vi "Vision Processing.vi"(4 "error in (no error)":errorcluster, 6 "CameraDevRef":T1) -> ()   [LabVIEW 2011]
uses:
  <vilib>/Rock Robotics/WPI/Camera/WPI_CameraDevRef.ctl
  Robot Global Data.vi
  <vilib>/vision/NI_Vision_Development_Module.lvlib
panel:
  in  "Default Shooter Speed Dump":dbl=0.42
  in  "Default Shooter Speed Shoot":dbl=0.705
  in  "Scale":dbl=0.85
  in  "Minimum Power":dbl=0.22
  out "Aspect Ratio":dbl[](array[numeric])
  out "Offset":dbl
  in  "Max Distance for 1 hoop":dbl=8.0
  out "Raw Turret":dbl
  in  "Run Calculations":bool=TRUE
  out "Target X Coord":dbl
  out "Target Distance":dbl
  out "Target Y Coord":dbl
  out "Distance Array":dbl[](array[numeric])
  in  "Dead Band":dbl=0.09
  out "Number of Rectangles Visible":dbl
  out "Y Position Array":dbl[](array[numeric])
  out "X Position Array":dbl[](array[numeric])
  in  "View":bool
  out "Target Info":T2(array[cluster])
  in  "Area Size Limit":i32=444
  in  "Particle Count Limit":i32=8
  in  "Score Limits":T3={"Rect Coverage"=76.0, "Aspect Ratio"=40.0, "X Edge Strength"=40.0, "Y Edge Strength"=60.0}
  in  "Processing":enum32{"Color", "Intensity", "Intensity Open"}(tab)=enum."Intensity"
  in  "Luminance":i32=255
  in  "Saturation":i32=255
  in  "Hue":i32(knob)=65 scale=0.0..255.0
  in  "Margins":cluster{"Hue":i32, "Sat":i32, "Lum":i32}={"Hue"=20, "Sat"=27, "Lum"=30} {"Sat" scale=0.0..40.0; "Lum" scale=0.0..40.0; "Hue" scale=0.0..40.0}
  in  "Range":cluster{"Lower value":sgl, "Upper value":sgl}={"Lower value"=151.52174, "Upper value"=255.0} {"Lower value" scale=0.0..255.0; "Upper value" scale=0.0..255.0}
  in  "Range":cluster{"Lower value":sgl, "Upper value":sgl}={"Lower value"=123.804344, "Upper value"=255.0} {"Lower value" scale=0.0..255.0; "Upper value" scale=0.0..255.0}
  in  "View":bool
  out "Processed Image":T4(plugin-control)
  out "Original Image":T4(plugin-control)
  # "Instructions:\nProcessing the reflective tape that is illuminated by a ring light can be based\non color or light intensity.\nParticles within the image are scored by rectangle coverage, aspect ratio, and\nfor being hollow with a bold edge. A particle is considered a target if all scores\nare above the score limits. Particles can be annotated -- surrounded by\na rectangle and scores drawn to the left .\nTo control the number of particles being scored, use the count limit and the size\nlimit."
  # "(in)"
  # "To debug, Enable using the View button.\nFor color processing, you can click in the image to select the color for processing."
  # "Enable by clicking the View button.\nGreen scores are above the limit, orange are below. Inner/outer rect\nindicates all passed."
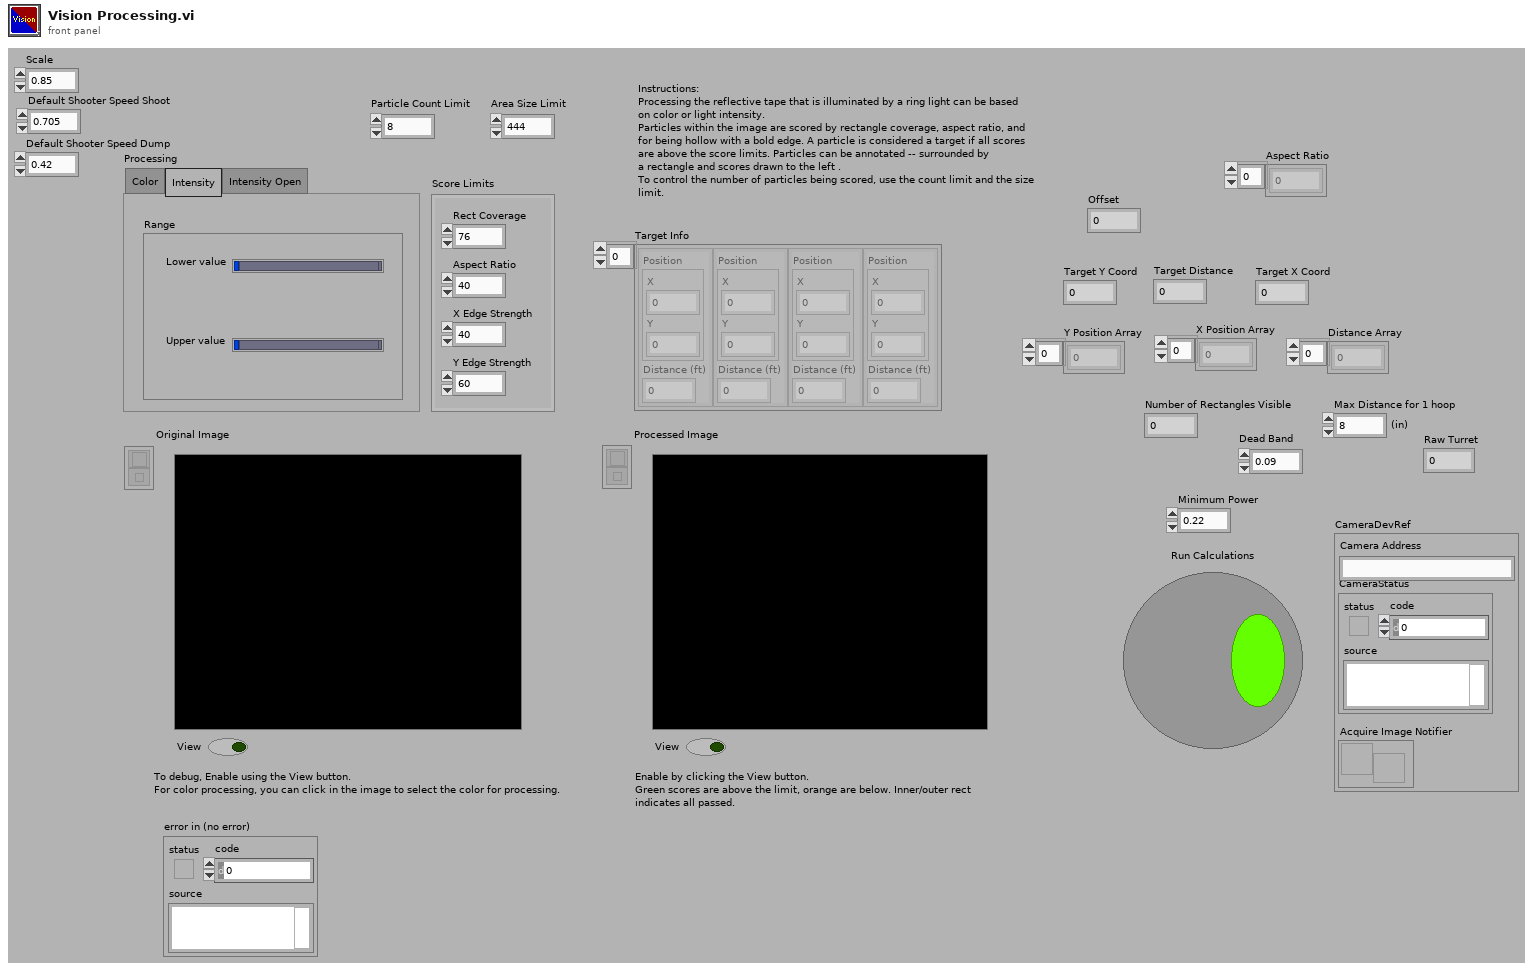
[diagram p1: front panel]
types:
  T1 = typedef "WPI_CameraDevRef.ctl" = cluster{"Camera Address":string, "CameraStatus":errorcluster, "Acquire Image Notifier":refnum<notifier>}
  T2 = cluster{"Position":cluster{"X":dbl, "Y":dbl}, "Distance (ft)":dbl}[]
  T3 = cluster{"Rect Coverage":dbl, "Aspect Ratio":dbl, "X Edge Strength":dbl, "Y Edge Strength":dbl}
  T4 = typedef "IMAQ Image.ctl" = refnum<image>
  T5 = typedef "Image Type" = u32
  T6 = enum32{"AutoM", "Close", "Dilate", "Erode", "Gradient", "Gradient out", "Gradient in", "Hit miss", "Open", "PClose", "POpen", "Thick", "Thin"}
  T7 = typedef "WPI_CameraImageSize.ctl" = enum16{"640x480", "320x240", "160x120"}
  T8 = cluster{"fps":i32, "compression":i32, "Image Size":T7}
  T9 = cluster{cluster{"Left":dbl, "Top":dbl, "Right":dbl, "Bottom":dbl}, dbl[]}[]
  T10 = cluster{"Left":dbl, "Top":dbl, "Right":dbl, "Bottom":dbl}
  T11 = cluster{"Target Center (-1 to 1)":cluster{"X":dbl, "Y":dbl}, "Distance (ft)":dbl}
  T12 = cluster{"Target Center (-1 to 1)":cluster{"X":dbl, "Y":dbl}, "Distance (ft)":dbl}[]
  T13 = typedef "WPI_JoystickDevRef.ctl" = cluster{"Device":T14}
  T14 = typedef "WPI_JoystickDeviceEnum.ctl" = enum16{"USB 1", "USB 2", "USB 3", "USB 4", "Kinect 1", "Kinect 2"}
  T15 = typedef "WPI_JoystickButtonState.ctl" = cluster{"Button 1":bool, "Button 2":bool, "Button 3":bool, "Button 4":bool, "Button 5":bool, "Button 6":bool, "Button 7":bool, "Button 8":bool, "Button 9":bool, "Button 10":bool, "Button 11":bool, "Button 12":bool}
  T16 = cluster{"axis 1 (x)":dbl, "axis 2 (y)":dbl, "axis 3 (throttle)":dbl, "axis 4":dbl, "axis 5":dbl, "axis 6":dbl}
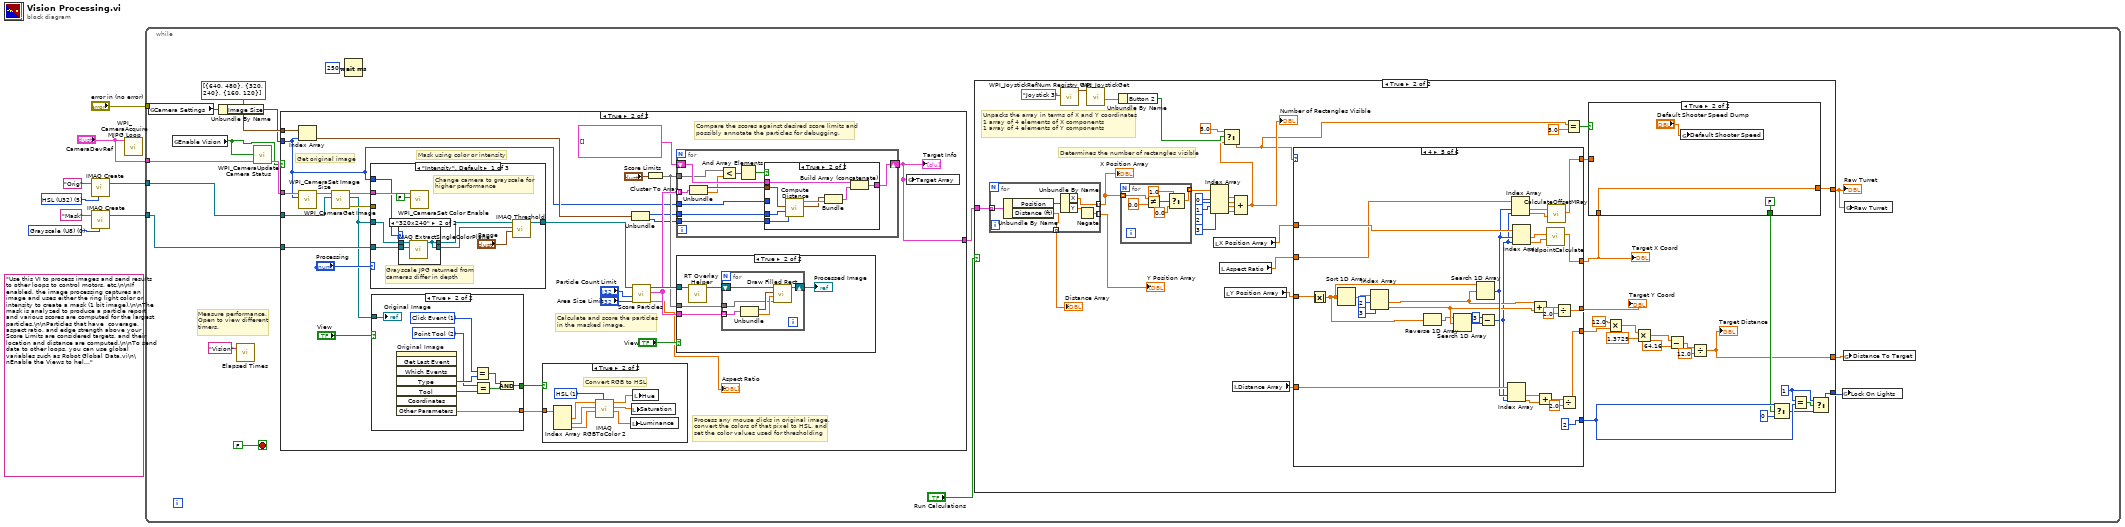
[diagram p0: block diagram]
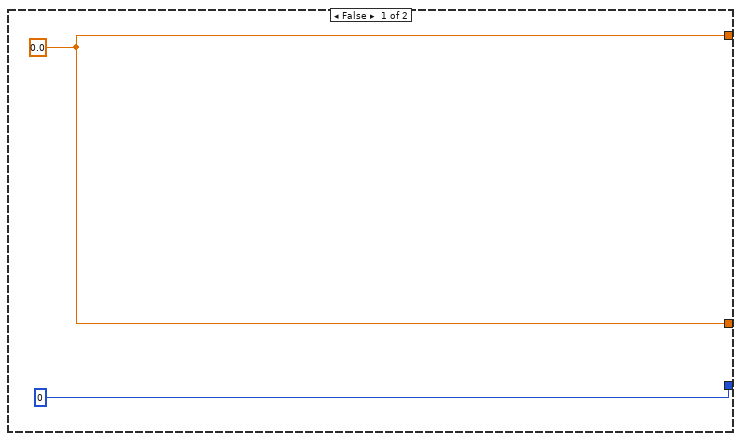
[diagram p2: hidden frame]
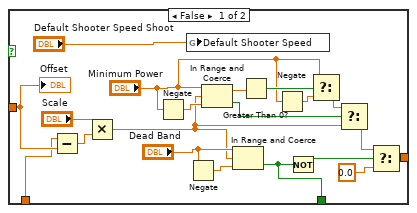
[diagram p3: hidden frame]
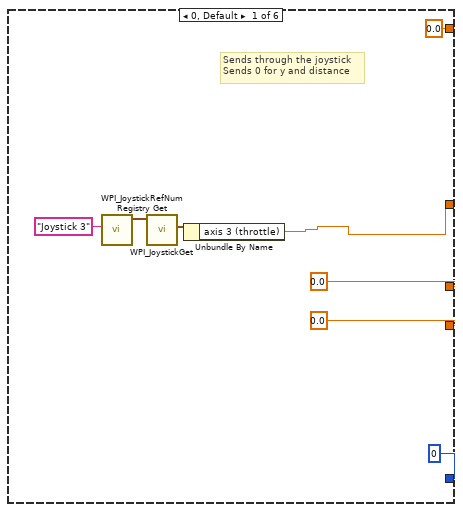
[diagram p4: hidden frame]
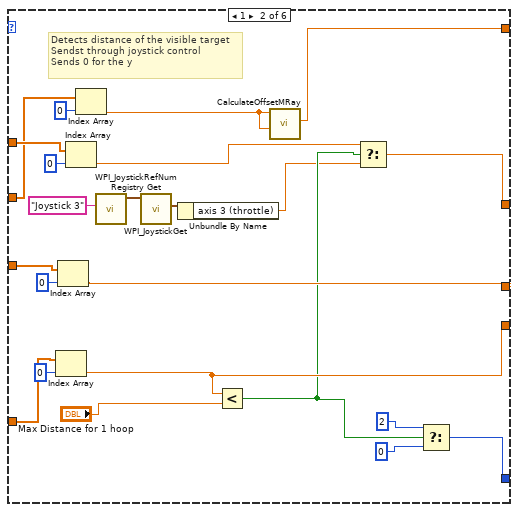
[diagram p5: hidden frame]
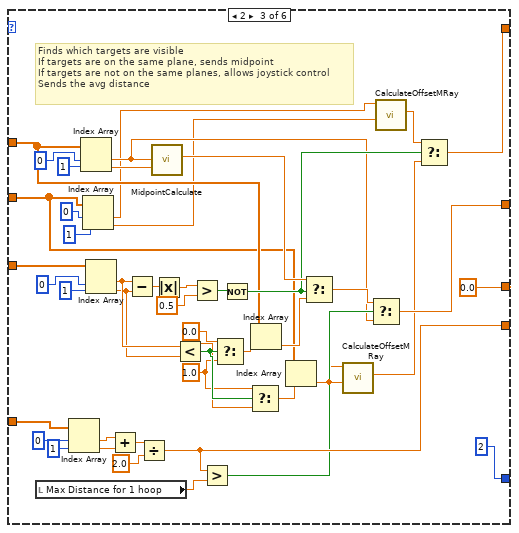
[diagram p6: hidden frame]
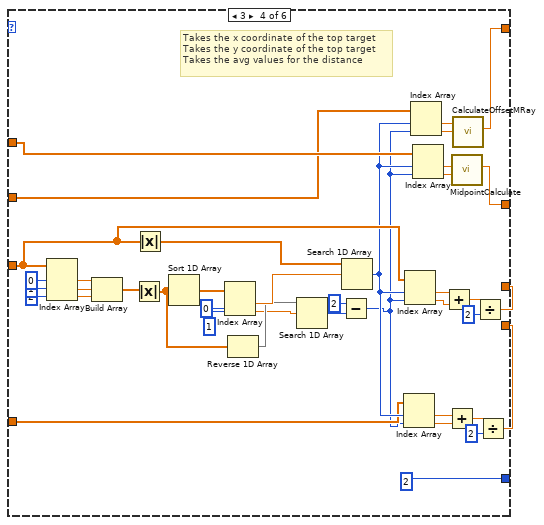
[diagram p7: hidden frame]
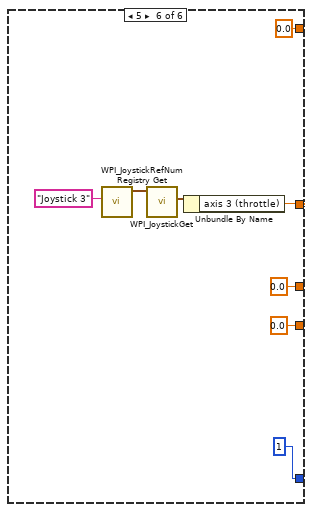
[diagram p8: hidden frame]
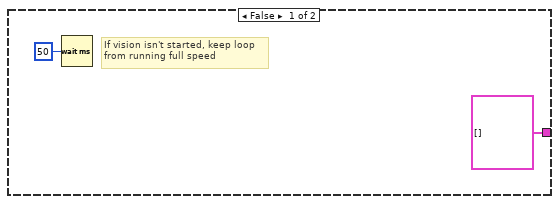
[diagram p9: hidden frame]
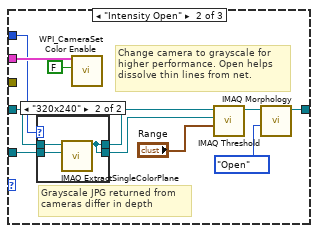
[diagram p12: hidden frame]
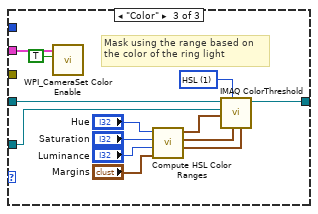
[diagram p14: hidden frame]
diagram:
  w3 = T5 0 items=["Grayscale (U8)", "Grayscale (I16)", "Grayscale (SGL)", "Complex (CSG)", "RGB (U32)", "HSL (U32)", "RGB (U64)", "Grayscale (U16)"] ("Image Type")
  (unwired) "Use this VI to process images and send results to other loops to control motors, etc.\n\nIf enabled, the image processing captures an image and uses either the ring light color or intensity to create a mask (1 bit image).\n\nThe mask is analyzed to produce a particle report and various scores are computed for the largest particles.\n\nParticles that have  coverage, aspect ratio, and edge strength above your Score Limits are considered targets, and their location and distance are computed.\n\nTo send data to other loops, you can use global variables such as Robot Global Data.vi\n\nEnable the Views to help debug color settings. Disable the View to speed up processing."
  w7 = T5 5 items=["Grayscale (U8)", "Grayscale (I16)", "Grayscale (SGL)", "Complex (CSG)", "RGB (U32)", "HSL (U32)", "RGB (U64)", "Grayscale (U16)"] ("Image Type")
  n1 = call "IMAQ Create"("Image Name"="Orig", "Image Type"=w7) -> ("New Image"=w6:T4)  [unwired: 2 in, 2 out]
  n2 = call "IMAQ Create"("Image Name"="Mask", "Image Type"=w3) -> ("New Image"=w1:T4)  [unwired: 2 in, 2 out]
  n3 = call <vilib>:"WPI_CameraAcquire MJPG Loop.vi"("CameraDevRef"="CameraDevRef") -> ()  [unwired: 11 in]
  n4 = while {
    tunnel: w6 -> [w23]
    tunnel: "CameraDevRef" -> [w22]
    tunnel: "error in (no error)" -> [_]
    tunnel: w1 -> [w18]
    stop <- FALSE stop-if-true
    # "Measure performance.\nOpen to view different\ntimers."
    n5 = global read "Robot Global Data.vi" "Camera Settings"() -> (w16:T8)
    n6 = global read "Robot Global Data.vi" "Enable Vision"() -> (w20:bool)
    n7 = Unbundle By Name(w16) -> ("Image Size"=w15:T7)
    n8 = call "Elapsed Times.vi"("Call Name"="Vision") -> ()  [unwired: 2 in, 1 out]
    n9 = call <vilib>:"WPI_CameraUpdate Camera Status.vi"("CameraDevRef In"=w22, "Enable Vision"=w20) -> ("CameraDevRef Out"=w21:T1)  [unwired: 3 in]
    n10 = case shown="True" w20 {
      tunnel: w23 -> [_ w281]
      tunnel: w21 -> [_ w277]
      tunnel: w18 -> [_ w268]
      tunnel: cluster{i32, i32}[] [{640, 480}, {320, 240}, {160, 120}] -> [_ w272]
      tunnel: w15 -> [_ w265]
      tunnel: [T2 [] w266] -> w14
      frame False {
        # "If vision isn't started, keep loop\nfrom running full speed"
        n11 = Wait (ms)(milliseconds to wait=u32 50) -> ()  [unwired: 1 out]
      }
      frame True {
        # "Compare the scores against desired score limits and\npossibly annotate the particles for debugging."
        # "Process any mouse clicks in original image,\nconvert the colors of that pixel to HSL, and\nset the color values used for thresholding"
        # "Calculate and score the particles\nin the masked image."
        # "Mask using color or intensity"
        # "Get original image"
        n12 = call <vilib>:"WPI_CameraSet Image Size.vi"("Image Size"=w265, "CameraDevRef"=w277) -> ("CameraDevRef Out"=w278:T1)  [unwired: 8 in, 1 out]
        n13 = Index Array(array=w272, index=w265) -> (element=w269:cluster{i32, i32})
        n14 = call <vilib>:"WPI_CameraGet Image.vi"("Image"=w281, "CameraDevRef"=w278) -> ("error out"=w279:errorcluster, "Image Out"=w267:T4, "CameraDevRef Out"=w280:T1)  [unwired: 7 in]
        n15 = case shown="\"Intensity\", Default" "Processing" {
          tunnel: w267 -> [w303 w315 w341]
          tunnel: [w306 w320 w340] -> w275
          tunnel: w280 -> [w304 w318 w331]
          tunnel: w279 -> [_ _ _]
          tunnel: w268 -> [w302 w316 w329]
          tunnel: w265 -> [w301 w317 _]
          frame "Intensity", Default {
            # "Grayscale JPG returned from\ncameras differ in depth"
            # "Change camera to grayscale for\nhigher performance"
            n16 = case shown="\"320x240\"" w301 {
              tunnel: w303 -> [w309 w312]
              tunnel: w302 -> [w308 w311]
              tunnel: [w309 w310] -> w300
              tunnel: [w308 w310] -> w299
              frame "640x480", Default {
              }
              frame "320x240" {
                n17 = call "IMAQ ExtractSingleColorPlane"("Image Dst"=w311, "Image Src"=w312) -> ("Image Dst Out"=w310:T4)  [unwired: 8 in, 1 out]
              }
            }
            n18 = call <vilib>:"WPI_CameraSet Color Enable.vi"("Color Enabled"=FALSE, "CameraDevRef"=w304) -> ()  [unwired: 8 in, 2 out]
            n19 = call "IMAQ Threshold"("Range"="Range", "Image Dst"=w299, "Image Src"=w300) -> ("Image Dst Out"=w306:T4)  [unwired: 3 in, 5 out]
          }
          frame "Intensity Open" {
            # "Grayscale JPG returned from\ncameras differ in depth"
            # "Change camera to grayscale for\nhigher performance. Open helps\ndissolve thin lines from net."
            n20 = case shown="\"320x240\"" w317 {
              tunnel: w315 -> [w325 w328]
              tunnel: w316 -> [w324 w327]
              tunnel: [w325 w326] -> w314
              tunnel: [w324 w326] -> w313
              frame "640x480", Default {
              }
              frame "320x240" {
                n21 = call "IMAQ ExtractSingleColorPlane"("Image Dst"=w327, "Image Src"=w328) -> ("Image Dst Out"=w326:T4)  [unwired: 8 in, 1 out]
              }
            }
            n22 = call <vilib>:"WPI_CameraSet Color Enable.vi"("Color Enabled"=FALSE, "CameraDevRef"=w318) -> ()  [unwired: 8 in, 2 out]
            n23 = call "IMAQ Threshold"("Range"="Range", "Image Dst"=w313, "Image Src"=w314) -> ("Image Dst Out"=w321:T4)  [unwired: 3 in, 5 out]
            n24 = call "IMAQ Morphology"("Operation"=T6."Open", "Image Src"=w321) -> ("Image Dst Out"=w320:T4)  [unwired: 8 in, 1 out]
          }
          frame "Color" {
            w339 = u16 1 items=["RGB", "HSL", "HSV", "HSI"] ("Color Mode")
            # "Mask using the range based on\nthe color of the ring light"
            n25 = call <vilib>:"WPI_CameraSet Color Enable.vi"("Color Enabled"=TRUE, "CameraDevRef"=w331) -> ()  [unwired: 8 in, 2 out]
            n26 = call "Compute HSL Color Ranges.vi"("Margins"="Margins", "Luminance"="Luminance", "Saturation"="Saturation", "Hue"="Hue") -> ("Lum Range"=w336:cluster{i32, i32}, "Sat Range"=w337:cluster{i32, i32}, "Hue Range"=w338:cluster{i32, i32})  [unwired: 5 in]
            n27 = call "IMAQ ColorThreshold"("Blue or Luma or Val or Inten Range"=w336, "Green or Sat Range"=w337, "Color Mode"=w339, "Red or Hue Range"=w338, "Image Dst"=w329, "Image Src"=w341) -> ("Image Dst Out"=w340:T4)  [unwired: 4 in, 1 out]
          }
        }
        n28 = case shown="True" "View" {
          tunnel: w267 -> [_ w361]
          tunnel: [_ w356] -> w274
          tunnel: [_ w353] -> w273
          frame False {
          }
          frame True {
            w354 = 2 items=["None", "Selection Tool", "Point Tool", "Line Tool", "Rectangle Tool", "Oval Tool", "Polygon Tool", "ClosedFreehandTool", "Annulus Tool", "Rotated Rectangle Tool", "Zoom Tool", "Pan Tool", "Polyline Tool", "Freehand Tool"] ("Tool")
            w355 = 1 items=["No Event"=0, "Click Event"=1, "Draw Event"=2, "Size Event"=4, "Scroll Event"=5, "Double Click Event"=8] ("Type")
            n29 = invoke on="Original Image" class="ImageControl" method="Get Last Event"() -> ("Type"=w357:i32, "Tool"=w360:i32, "Other Parameters"=w353:sgl[])  [unwired: 8 in, 5 out]
            n30 = Equal?(x=w355, y=w357) -> (x = y?=w358:bool)
            n31 = Equal?(x=w354, y=w360) -> (x = y?=w359:bool)
            n32 = And(x=w358, y=w359) -> (x .and. y?=w356:bool)
            "Original Image" <- w361
          }
        }
        n33 = case shown="True" w274 {
          tunnel: w273 -> [_ w298]
          frame False {
          }
          frame True {
            w297 = u16 1 items=["RGB", "HSL", "HSV", "HSI", "CIE L*a*b*", "CIE XYZ"] ("Color Mode")
            # "Convert RGB to HSL"
            n34 = Index Array(array=w298) -> (element #1=w296:sgl, element #2=w294:sgl, element #3=w292:sgl)  [unwired: 3 in]
            n35 = call "IMAQ RGBToColor 2"("Color Mode"=w297, "Blue value"=w292, "Green value"=w294, "Red value"=w296) -> ("Blue or Luma or Val or Inten or Z or b*value"=w291:dbl, "Green or Sat or Y or a* value"=w293:dbl, "Red or Hue or X or L* value"=w295:dbl)  [unwired: 4 in, 1 out]
            n36 = local write "Luminance"(w291) -> ()
            n37 = local write "Saturation"(w293) -> ()
            n38 = local write "Hue"(w295) -> ()
          }
        }
        n39 = Unbundle(w269) -> (w271:i32, w270:i32)
        n40 = call "Score Particles.vi"("Area Size Limit"="Area Size Limit", "Particle Count Limit"="Particle Count Limit", "Image Refnum in"=w275) -> ("Aspect Ratio"=→"Aspect Ratio":dbl[], "Scored Particle Info"=w286:T9, "Image Refnum out"=w289:T4)  [unwired: 6 in]
        n41 = Cluster To Array(cluster="Score Limits") -> (array=w284:dbl[])
        n42 = for {
          shift-right: [w371] -> w266
          shift-left: T2 [] -> [w372]
          tunnel: w271 -> [w370]
          tunnel: w286 -> [w368] mode=indexing
          tunnel: w284 -> [w363]
          tunnel: w265 -> [w367]
          tunnel: w270 -> [w362]
          n43 = Unbundle(w368) -> (w369:T10, w364:dbl[])
          n44 = Less?(x=w363, y=w364) -> (x < y?=w366:bool[])
          n45 = And Array Elements(Boolean array=w366) -> (logical AND=w365:bool)
          n46 = case shown="True" w365 {
            tunnel: w372 -> [w373 w381]
            tunnel: [w373 w380] -> w371
            tunnel: w369 -> [_ w376]
            tunnel: w370 -> [_ w378]
            tunnel: w367 -> [_ _]
            tunnel: w362 -> [_ w375]
            frame False {
            }
            frame True {
              n47 = call "Compute Distance.vi"("Y Image Resolution"=w375, "X Image Resolution"=w378, "Bounding Box"=w376) -> ("Target Center (-1 to 1)"=w374:cluster{"X":dbl, "Y":dbl}, "Distance (ft)"=w377:dbl)  [unwired: 7 in]
              n48 = Bundle("Target Center (-1 to 1)"=w374, "Distance (ft)"=w377) -> (w379:T11)  [unwired: 1 in]
              n49 = Build Array (concatenate)(w381, w379) -> (w380:T12)
            }
          }
        }
        "Target Info" <- w266
        n50 = case shown="True" "View" {
          tunnel: w289 -> [_ w343]
          tunnel: w286 -> [_ w345]
          tunnel: w284 -> [_ w344]
          frame False {
          }
          frame True {
            n51 = call "RT Overlay Helper.vi"("Refnum in"=w343) -> ("Refnum out"=w346:T4)  [unwired: 10 in]
            n52 = for {
              shift-right: [w351] -> w342
              shift-left: w346 -> [w352]
              tunnel: w345 -> [w348] mode=indexing
              tunnel: w344 -> [w347]
              n53 = Unbundle(w348) -> (w349:T10, w350:dbl[])
              n54 = call "Draw Filled Rect.vi"("Limits"=w347, "Scores"=w350, "Bounding Box"=w349, "image in"=w352) -> ("image out"=w351:T4)  [unwired: 7 in]
            }
            "Processed Image" <- w342
          }
        }
        n55 = global write "Robot Global Data.vi" "Target Array"(w266) -> ()
      }
    }
    n56 = Wait (ms)(milliseconds to wait=u32 250) -> ()  [unwired: 1 out]
    n57 = case shown="True" "Run Calculations" {
      tunnel: w14 -> [_ w55]
      tunnel: [w25 w37] -> w11
      tunnel: [0 ("f") w48] -> w10
      tunnel: [w25 w31] -> w9
      frame False {
        w25 = 0.0 ("f")
      }
      frame True {
        w49 = 1 ("y")
        # "Determines the number of rectangles visible"
        # "Unpacks the array in terms of X and Y coordinates\n1 array of 4 elements of X components\n1 array of 4 elements of Y components"
        n58 = for {
          tunnel: [w259] -> w56 mode=indexing
          tunnel: [w260] -> w66 mode=indexing
          tunnel: w55 -> [w257] mode=indexing
          tunnel: [w256] -> w68 mode=indexing
          n59 = Unbundle By Name(w257) -> ("Position"=w261:cluster{"X":dbl, "Y":dbl}, "Distance (ft)"=w256:dbl)
          n60 = Unbundle By Name(w261) -> ("X"=w260:dbl, "Y"=w258:dbl)
          n61 = Negate(x=w258) -> (-x=w259:dbl)
        }
        "X Position Array" <- w66
        "Y Position Array" <- w56
        "Distance Array" <- w68
        n62 = call <vilib>:"WPI_JoystickRefNum Registry Get.vi"("refnum name"="Joystick 3") -> ("JoystickDevRef"=w54:T13)  [unwired: 9 in, 1 out]
        n63 = call <vilib>:"WPI_JoystickGet.vi"("JoystickDevRef"=w54) -> ("Buttons"=w52:T15)  [unwired: 4 in, 2 out]
        n64 = Unbundle By Name(w52) -> ("Button 2"=w51:bool)
        n65 = for {
          tunnel: w66 -> [w100] mode=indexing
          tunnel: [w96] -> w65 mode=indexing
          n66 = Not Equal?(x=w100, y=0.0) -> (x != y?=w99:bool)
          n67 = Select(t=1.0, s=w99, f=0.0) -> (s? t:f=w96:dbl)
        }
        n68 = Index Array(array=w65, index #1=0 ("index"), index #2=1 ("index"), index #3=2 ("index"), index #4=3 ("index")) -> (element #1=w63:dbl, element #2=w64:dbl, element #3=w62:dbl, element #4=w61:dbl)
        n69 = local read "X Position Array"() -> (w67:dbl[])
        n70 = local read "Aspect Ratio"() -> (w43:dbl[])
        n71 = local read "Y Position Array"() -> (w70:dbl[])
        n72 = local read "Distance Array"() -> (w71:dbl[])
        n73 = Compound Arithmetic op=ADD(w63, w64, w62, w61) -> (w44:dbl)
        "Number of Rectangles Visible" <- w44
        n74 = Select(t=5.0, s=w51, f=w44) -> (s? t:f=w27:dbl)
        n75 = case shown="4" w27 {
          tunnel: w67 -> [_ w129 w141 w203 w243 _]
          tunnel: [w103 w123 w151 w184 w239 w249] -> w41
          tunnel: [0.0 ("X") w120 0.0 ("X") w204 w238 0.0 ("X")] -> w69
          tunnel: [0.0 ("X") w125 w154 w194 w233 0.0 ("X")] -> w35
          tunnel: w70 -> [_ w121 w175 w199 w247 _]
          tunnel: w71 -> [_ w132 w163 w186 w242 _]
          tunnel: [0 w116 2 2 2 1] -> w47
          tunnel: [0.0 ("Offset") w113 w138 w191 w229 0.0 ("Offset")] -> w42
          tunnel: w43 -> [_ w112 w133 w187 w225 _]
          frame 0, Default {
            # "Sends through the joystick\nSends 0 for y and distance"
            n76 = call <vilib>:"WPI_JoystickRefNum Registry Get.vi"("refnum name"="Joystick 3") -> ("JoystickDevRef"=w107:T13)  [unwired: 9 in, 1 out]
            n77 = call <vilib>:"WPI_JoystickGet.vi"("JoystickDevRef"=w107) -> ("Axes"=w105:T16)  [unwired: 4 in, 2 out]
            n78 = Unbundle By Name(w105) -> ("axis 3 (throttle)"=w103:dbl)
          }
          frame 1 {
            # "Detects distance of the visible target\nSendst through joystick control\nSends 0 for the y"
            n79 = Index Array(array=w132, index=0) -> (element=w125:dbl)
            n80 = Index Array(array=w121, index=0) -> (element=w120:dbl)
            n81 = Index Array(array=w129, index=0) -> (element=w114:dbl)
            n82 = Index Array(array=w112, index=0) -> (element=w110:dbl)
            n83 = call <vilib>:"WPI_JoystickRefNum Registry Get.vi"("refnum name"="Joystick 3") -> ("JoystickDevRef"=w128:T13)  [unwired: 9 in, 1 out]
            n84 = call <vilib>:"WPI_JoystickGet.vi"("JoystickDevRef"=w128) -> ("Axes"=w126:T16)  [unwired: 4 in, 2 out]
            n85 = Unbundle By Name(w126) -> ("axis 3 (throttle)"=w115:dbl)
            n86 = Less?(x=w125, y="Max Distance for 1 hoop") -> (x < y?=w118:bool)
            n87 = call "CalculateOffsetMRay.vi"("AR2"=w110, "AR1"=w110) -> ("Offset"=w113:dbl)  [unwired: 9 in]
            n88 = Select(t=w114, s=w118, f=w115) -> (s? t:f=w123:dbl)
            n89 = Select(t=2, s=w118, f=0) -> (s? t:f=w116:i32)
          }
          frame 2 {
            w144 = 1.0 ("f")
            w143 = 0.0 ("t")
            # "Finds which targets are visible\nIf targets are on the same plane, sends midpoint\nIf targets are not on the same planes, allows joystick control\nSends the avg distance"
            n90 = local read "Max Distance for 1 hoop"() -> (w153:dbl)
            n91 = Index Array(array=w163, index #1=0 ("index"), index #2=1 ("index")) -> (element #1=w162:dbl, element #2=w161:dbl)
            n92 = Index Array(array=w141, index #1=0 ("index"), index #2=1 ("index")) -> (element #1=w148:dbl, element #2=w147:dbl)
            n93 = Index Array(array=w133, index #1=0 ("index"), index #2=1 ("index")) -> (element #1=w135:dbl, element #2=w134:dbl)
            n94 = Index Array(array=w175, index #1=0 ("index"), index #2=1 ("index")) -> (element #1=w159:dbl, element #2=w158:dbl)
            n95 = Add(x=w162, y=w161) -> (x+y=w166:dbl)
            n96 = Subtract(x=w159, y=w158) -> (x-y=w172:dbl)
            n97 = Divide(x=w166, y=2.0) -> (x/y=w154:dbl)
            n98 = call "MidpointCalculate.vi"("X2"=w147, "X1"=w148) -> ("Midpoint"=w168:dbl)  [unwired: 9 in]
            n99 = Absolute Value(x=w172) -> (abs(x)=w171:dbl)
            n100 = Less?(x=w159, y=w158) -> (x < y?=w145:bool)
            n101 = Greater?(x=w171, y=0.5) -> (0:w169:bool)
            n102 = Greater?(x=w154, y=w153) -> (0:w152:bool)
            n103 = Select(t=w143, s=w145, f=w144) -> (s? t:f=w157:dbl)
            n104 = Not(x=w169) -> (.not. x?=w149:bool)
            n105 = Select(t=w144, s=w145, f=w143) -> (s? t:f=w142:dbl)
            n106 = Index Array(array=w141, index=w157) -> (element=w156:dbl)
            n107 = Index Array(array=w133, index=w142) -> (element=w140:dbl)
            n108 = Select(t=w168, s=w149, f=w156) -> (s? t:f=w150:dbl)
            n109 = call "CalculateOffsetMRay.vi"("AR2"=w140, "AR1"=w140) -> ("Offset"=w139:dbl)  [unwired: 9 in]
            n110 = Select(t=w150, s=w152, f=w148) -> (s? t:f=w151:dbl)
            n111 = call "CalculateOffsetMRay.vi"("AR2"=w134, "AR1"=w135) -> ("Offset"=w146:dbl)  [unwired: 9 in]
            n112 = Select(t=w146, s=w149, f=w139) -> (s? t:f=w138:dbl)
          }
          frame 3 {
            # "Takes the x coordinate of the top target\nTakes the y coordinate of the top target\nTakes the avg values for the distance"
            n113 = Index Array(array=w199, index #1=0 ("index"), index #2=1 ("index"), index #3=2 ("index")) -> (element #1=w214:dbl, element #2=w213:dbl, element #3=w212:dbl)
            n114 = Build Array(w214, w213, w212) -> (w211:dbl[])
            n115 = Absolute Value(x=w211) -> (abs(x)=w182:dbl[])
            n116 = Absolute Value(x=w199) -> (abs(x)=w202:dbl[])
            n117 = Sort 1D Array(array=w182) -> (sorted array=w210:dbl[])
            n118 = Index Array(array=w210, index #1=0 ("index"), index #2=1 ("index")) -> (element #1=w207:dbl, element #2=w180:dbl)
            n119 = Reverse 1D Array(array=w182) -> (reversed array=w181:dbl[])
            n120 = Search 1D Array(1D array=w181, element=w180) -> (index of element=w183:i32)  [unwired: 1 in]
            n121 = Subtract(x=2, y=w183) -> (x-y=w178:i32)
            n122 = Search 1D Array(1D array=w202, element=w207) -> (index of element=w190:i32)  [unwired: 1 in]
            n123 = Index Array(array=w186, index #1=w190, index #2=w178) -> (element #1=w196:dbl, element #2=w195:dbl)
            n124 = Index Array(array=w199, index #1=w190, index #2=w178) -> (element #1=w201:dbl, element #2=w200:dbl)
            n125 = Index Array(array=w187, index #1=w190, index #2=w178) -> (element #1=w189:dbl, element #2=w188:dbl)
            n126 = Index Array(array=w203, index #1=w190, index #2=w178) -> (element #1=w185:dbl, element #2=w192:dbl)
            n127 = Add(x=w201, y=w200) -> (x+y=w206:dbl)
            n128 = Add(x=w196, y=w195) -> (x+y=w197:dbl)
            n129 = call "MidpointCalculate.vi"("X2"=w192, "X1"=w185) -> ("Midpoint"=w184:dbl)  [unwired: 9 in]
            n130 = call "CalculateOffsetMRay.vi"("AR2"=w188, "AR1"=w189) -> ("Offset"=w191:dbl)  [unwired: 9 in]
            n131 = Divide(x=w206, y=2) -> (x/y=w204:dbl)
            n132 = Divide(x=w197, y=2) -> (x/y=w194:dbl)
          }
          frame 4 {
            n133 = Absolute Value(x=w247) -> (abs(x)=w221:dbl[])
            n134 = Sort 1D Array(array=w221) -> (sorted array=w246:dbl[])
            n135 = Index Array(array=w246, index #1=2 ("index"), index #2=3 ("index")) -> (element #1=w224:dbl, element #2=w223:dbl)
            n136 = Reverse 1D Array(array=w221) -> (reversed array=w222:dbl[])
            n137 = Search 1D Array(1D array=w222, element=w223) -> (index of element=w220:i32)  [unwired: 1 in]
            n138 = Search 1D Array(1D array=w221, element=w224) -> (index of element=w228:i32)  [unwired: 1 in]
            n139 = Subtract(x=3, y=w220) -> (x-y=w219:i32)
            n140 = Index Array(array=w242, index #1=w228, index #2=w219) -> (element #1=w235:dbl, element #2=w234:dbl)
            n141 = Index Array(array=w225, index #1=w228, index #2=w219) -> (element #1=w226:dbl, element #2=w227:dbl)
            n142 = Index Array(array=w243, index #1=w228, index #2=w219) -> (element #1=w231:dbl, element #2=w230:dbl)
            n143 = Add(x=w224, y=w223) -> (x+y=w241:dbl)
            n144 = Add(x=w235, y=w234) -> (x+y=w236:dbl)
            n145 = call "MidpointCalculate.vi"("X2"=w230, "X1"=w231) -> ("Midpoint"=w239:dbl)  [unwired: 9 in]
            n146 = call "CalculateOffsetMRay.vi"("AR2"=w227, "AR1"=w226) -> ("Offset"=w229:dbl)  [unwired: 9 in]
            n147 = Divide(x=w241, y=2.0) -> (x/y=w238:dbl)
            n148 = Divide(x=w236, y=2.0) -> (x/y=w233:dbl)
          }
          frame 5 {
            n149 = call <vilib>:"WPI_JoystickRefNum Registry Get.vi"("refnum name"="Joystick 3") -> ("JoystickDevRef"=w253:T13)  [unwired: 9 in, 1 out]
            n150 = call <vilib>:"WPI_JoystickGet.vi"("JoystickDevRef"=w253) -> ("Axes"=w251:T16)  [unwired: 4 in, 2 out]
            n151 = Unbundle By Name(w251) -> ("axis 3 (throttle)"=w249:dbl)
          }
        }
        "Target Y Coord" <- w69
        "Target X Coord" <- w41
        n152 = Equal?(x=w27, y=5.0) -> (x = y?=w29:bool)
        n153 = case shown="True" w29 {
          tunnel: w42 -> [w91 _]
          tunnel: w41 -> [w90 w95]
          tunnel: [w77 w95] -> w37
          tunnel: [w75 FALSE] -> w36
          frame False {
            n154 = Subtract(x=w90, y=w91) -> (x-y=w88:dbl)
            n155 = Multiply(x="Scale", y=w88) -> (x*y=w79:dbl)
            n156 = Negate(x="Minimum Power") -> (-x=w86:dbl)
            n157 = global write "Robot Global Data.vi" "Default Shooter Speed"("Default Shooter Speed Shoot") -> ()
            n158 = Negate(x="Dead Band") -> (-x=w92:dbl)
            n159 = In Range and Coerce(upper limit="Minimum Power", x=w79, lower limit=w86) -> (coerced(x)=w82:dbl, In Range?=w83:bool)
            n160 = In Range and Coerce(upper limit="Dead Band", x=w79, lower limit=w92) -> (In Range?=w75:bool)  [unwired: 1 out]
            n161 = Greater Than 0?(x=w82) -> (x > 0?=w81:bool)
            n162 = Negate(x="Minimum Power") -> (-x=w78:dbl)
            n163 = Not(x=w75) -> (.not. x?=w76:bool)
            n164 = Select(t="Minimum Power", s=w81, f=w78) -> (s? t:f=w80:dbl)
            n165 = Select(t=w80, s=w83, f=w79) -> (s? t:f=w84:dbl)
            n166 = Select(t=w84, s=w76, f=0.0) -> (s? t:f=w77:dbl)
            "Offset" <- w91
          }
          frame True {
            n167 = global write "Robot Global Data.vi" "Default Shooter Speed"("Default Shooter Speed Dump") -> ()
          }
        }
        n168 = Multiply(x=12.0, y=w35) -> (x*y=w34:dbl)
        n169 = Multiply(x=w34, y=1.3729) -> (x*y=w39:dbl)
        n170 = Subtract(x=w39, y=64.16) -> (x-y=w32:dbl)
        n171 = Divide(x=w32, y=12.0) -> (x/y=w31:dbl)
        "Target Distance" <- w31
        n172 = Select(t=w47, s=w36, f=0) -> (s? t:f=w45:i32)
        n173 = Equal?(x=w49, y=w47) -> (x = y?=w50:bool)
        n174 = Select(t=w49, s=w50, f=w45) -> (s? t:f=w48:i32)
      }
    }
    "Raw Turret" <- w11
    n175 = global write "Robot Global Data.vi" "Lock On Lights"(w10) -> ()
    n176 = global write "Robot Global Data.vi" "Distance To Target"(w9) -> ()
    n177 = global write "Robot Global Data.vi" "Raw Turret"(w11) -> ()
  }
